vi "AppliOffsetAnalogSig.vi"(4 "error in (no error)":errorcluster, 6 "WaveFormIN":waveform(dbl)[](graph), 7 "NomProjet":string) -> (0 "error out":errorcluster, 2 "WaveFormOUT":waveform(dbl)[](graph))   [LabVIEW 2017]
uses:
  <vilib>/Analysis/baseanly.llb/Mean (DBL).vi
  <vilib>/Waveform/WDTOps.llb/WDT Get Waveform Subset DBL.vi
  <vilib>/Analysis/NI_AALBase.lvlib
panel:
  out "Offset(unités phys)":dbl[](array[numeric])
  out "AutoZero?":bool[](array[boolean])
  out "VoieN":waveform(dbl)(graph)
  out "DebutVoieN":waveform(dbl)(graph)
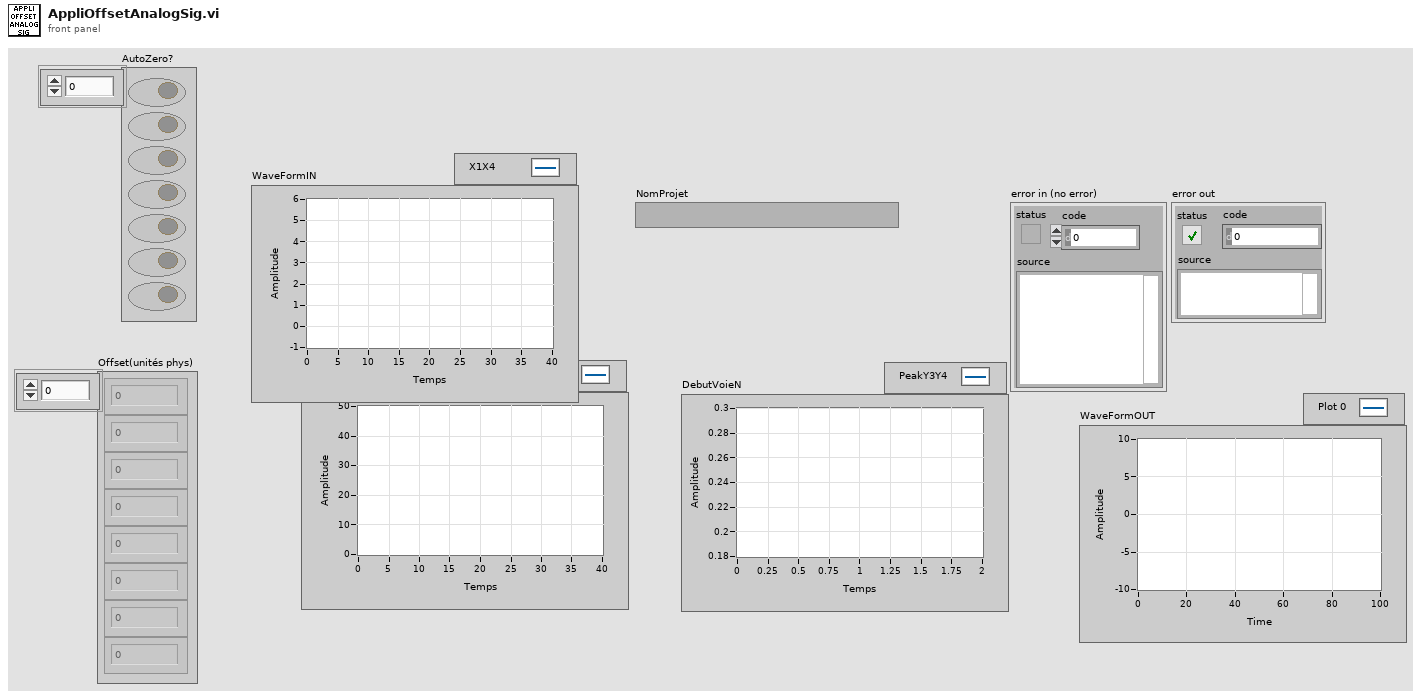
[diagram p1: front panel]
types:
  T1 = typedef "ConfigTotale.ctl" = cluster{"VoltageChannels":T2, "WheastoneBridgeChannels":T3, "Configuration":T4}
  T2 = typedef "VoltageChannels.ctl" = cluster{"ChannelNames":string[], "Sensitivity(Unit/V)":dbl[], "AutoZero":bool[], "ChannelUnits":string[], "Offsets(Units)":dbl[], "Graph Num":u8[]}
  T3 = typedef "WBridgeChannels.ctl" = cluster{"ChannelNames":string[], "Sensitivity(Unit/V)":dbl[], "AutoZero":bool[], "ChannelUnits":string[], "Offsets(Units)":dbl[], "Graph Num":u8[]}
  T4 = typedef "Configuration.ctl" = cluster{"AcqSamplingRate(Hz)":u32, "AcqTime(s)":u32, "Trigger":bool, "NbVoltageChannels":u32, "NbWBridgeChannels":u32, "Qualisys":bool, "Hexapode":bool, "FinalSamplingRate(Hz)":u32, "QualisysDataType":enum16{"6DOF", "3DTracking", "6DOF + 3D"}, "Nortek":bool, "HBM":bool}
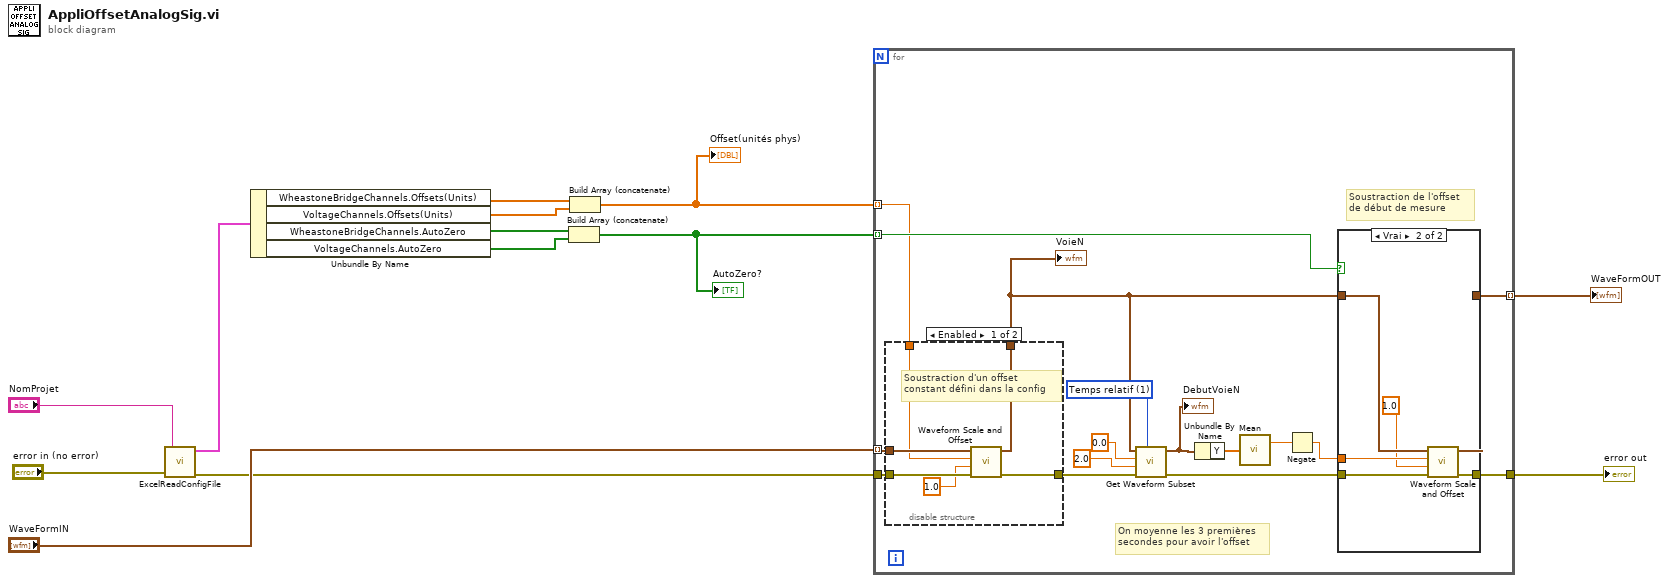
[diagram p0: block diagram]
diagram:
  n1 = call "ExcelReadConfigFile.vi"("NomProjet"="NomProjet", "error in (no error)"="error in (no error)") -> ("ConfigurationTotale"=w13:T1, "error out"=w3:errorcluster)  [unwired: 3 in]
  n2 = Unbundle By Name(w13) -> ("WheastoneBridgeChannels.Offsets(Units)"=w12:dbl[], "VoltageChannels.Offsets(Units)"=w11:dbl[], "WheastoneBridgeChannels.AutoZero"=w10:bool[], "VoltageChannels.AutoZero"=w9:bool[])
  n3 = Build Array (concatenate)(w10, w9) -> (w7:bool[])
  "AutoZero?" <- w7
  n4 = Build Array (concatenate)(w12, w11) -> (w8:dbl[])
  "Offset(unités phys)" <- w8
  n5 = for {
    tunnel: "WaveFormIN" -> [w17] mode=indexing
    tunnel: w7 -> [w29] mode=indexing
    tunnel: w3 -> [w19]
    tunnel: [w20] -> w2
    tunnel: [w21] -> w1 mode=indexing
    tunnel: w8 -> [w15] mode=indexing
    w26 = u16 1 items=["Échantillons", "Temps relatif"] ("start/duration format")
    # "Soustraction de l'offset \nde début de mesure"
    # "On moyenne les 3 premières\nsecondes pour avoir l'offset"
    n6 = disable-structure shown="Enabled" {
      disable-tunnel: w19 -> [w35 w36]
      disable-tunnel: [w34 w36] -> w18
      disable-tunnel: w17 -> [w33 w37]
      disable-tunnel: [w32 w37] -> w16
      disable-tunnel: w15 -> [w31 _]
      frame Enabled {
        # "Soustraction d'un offset\nconstant défini dans la config"
        n7 = call <vilib>:"Waveform Scale and Offset.vi"("error in (no error)"=w35, "scale"=1.0, "offset"=w31, "waveform in"=w33) -> ("error out"=w34:errorcluster, "waveform out"=w32:waveform(dbl))  [unwired: 6 in]
      }
      frame Disabled {
      }
    }
    "VoieN" <- w16
    n8 = call-poly <vilib>:"Get Waveform Subset.vi"("start/duration format"=w26, "error in (no error)"=w18, "duration"=2.0, "start samples/time"=0.0, "waveform in"=w16) -> ("error out"=w25:errorcluster, "waveform out"=w22:waveform(dbl))  [unwired: 1 in, 2 out]
    "DebutVoieN" <- w22
    n9 = Unbundle By Name(w22) -> ("Y"=w14:dbl[])
    n10 = call-poly <vilib>:"Mean.vi"("X"=w14) -> ("mean"=w23:dbl)  [unwired: 1 out]
    n11 = Negate(x=w23) -> (-x=w24:dbl)
    n12 = case shown="Vrai" w29 {
      tunnel: w24 -> [_ w44]
      tunnel: w16 -> [w39 w45]
      tunnel: w25 -> [w38 w42]
      tunnel: [w38 w41] -> w20
      tunnel: [w39 w40] -> w21
      frame False {
      }
      frame True {
        n13 = call <vilib>:"Waveform Scale and Offset.vi"("error in (no error)"=w42, "scale"=1.0, "offset"=w44, "waveform in"=w45) -> ("error out"=w41:errorcluster, "waveform out"=w40:waveform(dbl))  [unwired: 6 in]
      }
    }
  }
  "error out" <- w2
  "WaveFormOUT" <- w1
